vi "运维调试_五参数.vi"(11 "编号":string) -> ()   [LabVIEW 2016, in "斯坦道多参数.lvlib"]
uses:
  <vilib>/Utility/miscctls.llb/LVPointTypeDef.ctl
  <vilib>/Plasmionique/MB Master/MB_Master/MB_Master.lvclass
  <vilib>/Utility/config.llb/NI_LVConfig.lvlib
panel:
  in  "水样保存组数":dbl caption="水样保存组数:"
  in  "水样稳定时间":dbl caption="水样稳定时间:"
  in  "仪器参数":bool
  in  "参数设置选项卡":enum32{"选项卡 1", "选项卡 2"}(tab)
  in  "COD探头选择":u16(ring)=1 items=["YL型", "MQ型", "NAQ型"]
  in  "COD启用":bool
  in  "pH":bool
  in  "DO":bool
  in  "Turb":bool
  in  "Cond":bool
  in  "Temp":bool
  in  "叶绿素a启用":bool
  in  "藻密度":bool
  in  "pH探头选择":u16(ring) items=["YL型", "MQ型", "NAQ型"]
  in  "DO探头选择":u16(ring) items=["YL型", "MQ型", "NAQ型"]
  in  "电导率探头选择":u16(ring) items=["YL型", "MQ型", "NAQ型"]
  in  "浊度探头选择":u16(ring) items=["YL型", "MQ型", "NAQ型"]
  in  "叶绿素a探头选择":u16(ring) items=["YL型", "MQ型", "NAQ型"]
  in  "藻密度探头选择":u16(ring) items=["YL型", "MQ型", "NAQ型"]
  in  "ORP启用":bool
  in  "ORP探头选择":u16(ring) items=["YL型", "MQ型", "NAQ型"]
  in  "校准选择":T1
  out "模块版本号":string
  out "权限等级":string
  in  "打开modbus":bool
  out "选项卡控件":enum32{"选项卡 1", "选项卡 2"}(tab)
  in  "VISA资源名称":refnum<visa-resource-name> caption="串口"
  in  "IP":string="localhost" caption="IP:"
  in  "Port":u16=502 caption="Port:"
  in  "自动断线重连":bool=TRUE
  in  "连接方式":u16(ring) items=["Modbus RTU", "Modbus TCP"]
  in  "密码锁":bool
  in  "设置页返回":bool
  in  "周期设置":bool
  out "当前串口":string
  out "运行状态":enum16{"空闲", "水样测试", "标样核查"}(ring)
  in  "停止":bool
  in  "标样核查":bool
  in  "水样测试":bool
  in  "设置":bool
  in  "探头校正返回":bool
  in  "探头校正":bool
  out "检测值":T2
  # "请设置仪器连接方式"
  # "组"
  # "min"
  # "请选择要启用的参数"
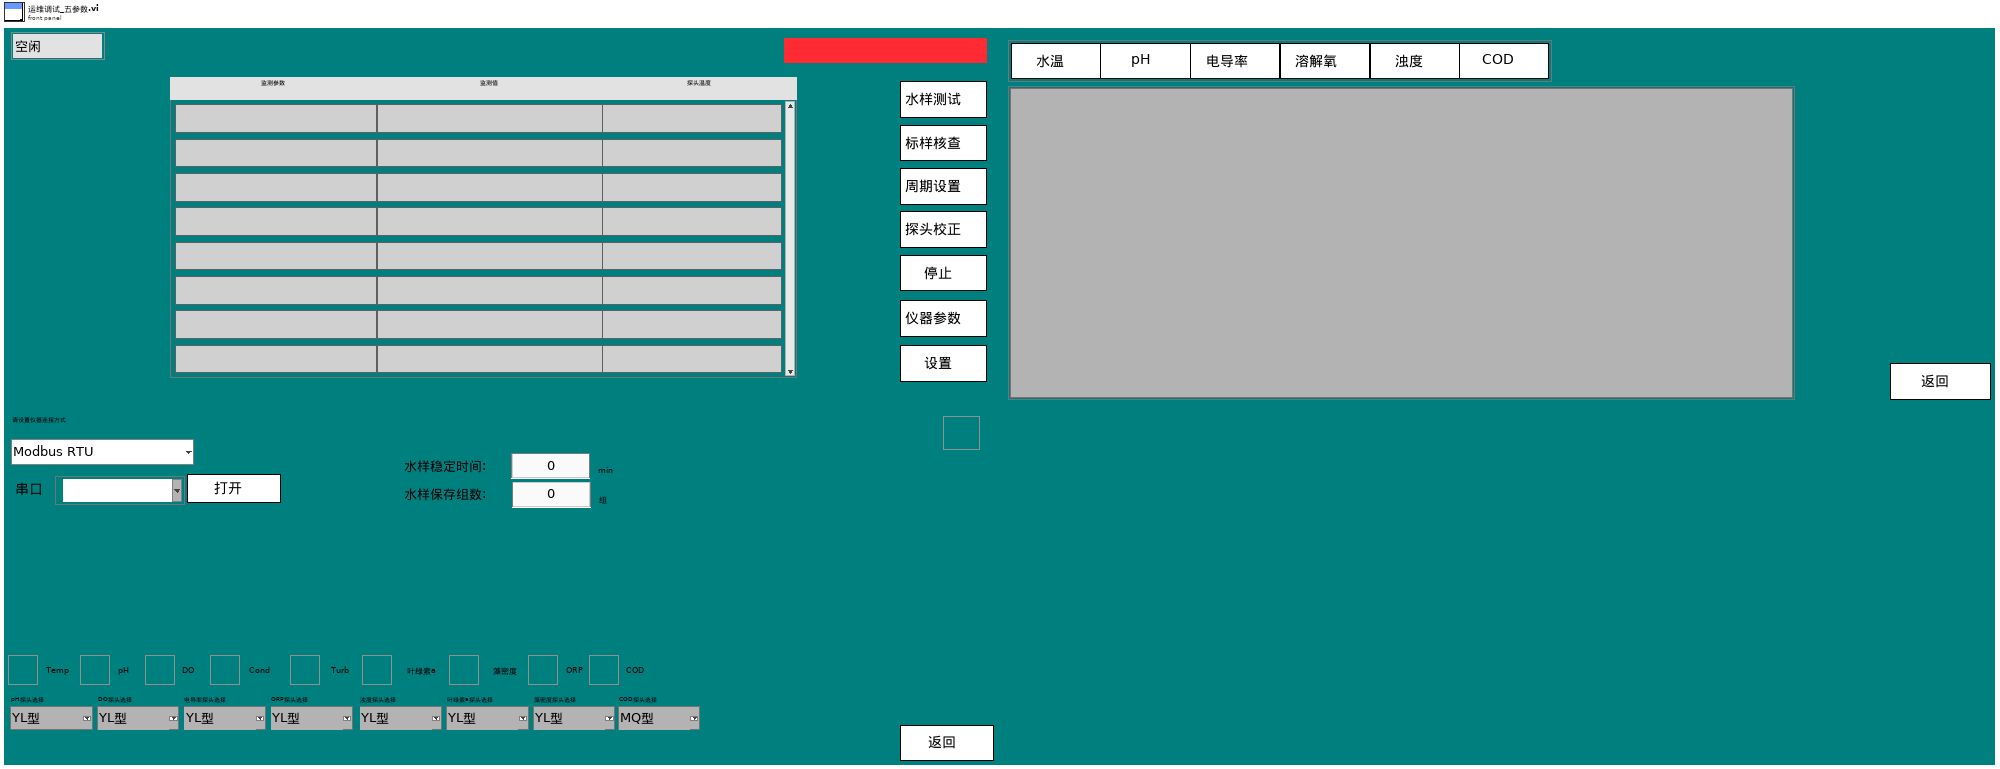
[diagram p1: front panel]
types:
  T1 = cluster{"水温校准":bool, "pH校准":bool, "电导率校准":bool, "溶解氧校准":bool, "浊度校准":bool, "叶绿素a校准":bool, "藻密度校准":bool, "ORP校准":bool, "COD校准":bool}
  T2 = typedef "斯坦道多参数.lvlib/检测值.ctl" = cluster{"监测参数1":string, "浓度1":string, "探头温度1":string}[]
  T3 = typedef "LVPointTypeDef.ctl" = cluster{"Horizontal":i16, "Vertical":i16}
  T4 = cluster{"CH":u16, "监测值":dbl, "温度偏移修正值":sgl, "信号值":sgl}
  T5 = cluster{"温度测量值":sgl, "测量值":sgl, "温度偏移修正值":sgl, "信号值":sgl}
  T6 = cluster{"温度测量值":sgl, "DO%":sgl, "DOmg/L":sgl, "温度偏移修正值":sgl}
  T7 = cluster{"电极状态标志":u16, "电极型号标志":u16, "浊度测量值":sgl, "温度测量值":sgl, "浊度信号值":sgl, "浊度偏移修正值":sgl, "温度偏移修正值":sgl, "手动温度补偿值":sgl, "浊度电极零点":sgl, "浊度电极斜率":sgl, "第1点标准值记录":sgl, "第1点信号值记录":sgl, "第1点温度值记录":sgl, "第2点标准值记录":sgl, "第2点信号值记录":sgl, "第2点温度值记录":sgl, "命令滤波设定":u16, "温度模式":enum16{"ATC", "MTC"}, "生产批次":u16, "电极序号":u16, "串口地址":u16, "串口波特率":enum16{"9600", "19200", "115200"}, "串口校验位":enum16{"NONE", "ODD", "EVEN"}, "串口停止位":enum16{"1bit", "2bit"}, "第一点标准值":sgl, "第二点标准值":sgl, "第三点标准值":sgl}
  T8 = cluster{"电极状态标志":u16, "电极型号标志":u16, "溶解氧测量值":sgl, "温度测量值":sgl, "溶解氧饱和度值":sgl, "盐度补偿值":sgl, "大气压补偿值":sgl, "溶解氧偏移修正值":sgl, "温度偏移修正值":sgl, "手动温度补偿值":sgl, "溶解氧电极零点":sgl, "溶解氧电极斜率":sgl, "第1点标准值记录":sgl, "第1点信号值记录":sgl, "第1点温度值记录":sgl, "第2点标准值记录":sgl, "第2点信号值记录":sgl, "第2点温度值记录":sgl, "命令滤波设定":u16, "温度模式":enum16{"ATC", "MTC"}, "生产批次":u16, "电极序号":u16, "串口地址":u16, "串口波特率":enum16{"9600", "19200", "115200"}, "串口校验位":enum16{"NONE", "ODD", "EVEN"}, "串口停止位":enum16{"1bit", "2bit"}, "第一点标准值":sgl, "第二点标准值":sgl}
  T9 = cluster{"电极状态标志":u16, "电极型号标志":u16, "酸碱度测量值":sgl, "温度测量值":sgl, "酸碱度信号值":sgl, "温度信号值":sgl, "酸碱度偏移修正值":sgl, "温度偏移修正值":sgl, "手动温度补偿值":sgl, "酸碱度电极零点":sgl, "酸碱度电极斜率":sgl, "第1点标准值记录":sgl, "第1点信号值记录":sgl, "第1点温度值记录":sgl, "第2点标准值记录":sgl, "第2点信号值记录":sgl, "第2点温度值记录":sgl, "命令滤波设定":u16, "温度模式":enum16{"ATC", "MTC"}, "生产批次":u16, "电极序号":u16, "串口地址":u16, "串口波特率":enum16{"9600", "19200", "115200"}, "串口校验位":enum16{"NONE", "ODD", "EVEN"}, "串口停止位":enum16{"1bit", "2bit"}, "第一点标准值":sgl, "第二点标准值":sgl}
  T10 = cluster{"测量量程":dbl, "测量精度":dbl, "测量间隔":dbl, "消解温度":dbl, "消解时长":dbl, "空白校准时间":timestamp, "曲线截距":dbl, "曲线斜率":dbl, "测量检出限":dbl, "测量信号值":dbl, "线性相关系数":dbl, "二次多项式系数":dbl, "标样校准时间":timestamp, "稀释倍数":dbl, "三项式系数":dbl, "空白标定系数":dbl, "量程系数":dbl, "F0/ORPA":dbl, "F1/ORPB":dbl, "F2/ORPK":dbl, "F3":dbl, "F4":dbl, "F5":dbl, "F6":dbl, "F7":dbl, "X0/滴定数":dbl, "量程":dbl}
  T11 = cluster{"电极状态标志":u16, "电极型号标志":u16, "电导率测量值":sgl, "温度测量值":sgl, "电导率信号值":sgl, "温度信号值":sgl, "温度补偿系数":sgl, "电导率偏移修正值":sgl, "温度偏移修正值":sgl, "手动温度补偿值":sgl, "电导率电极零点":sgl, "电导率电极斜率":sgl, "命令滤波设定":u16, "温度模式":enum16{"ATC", "MTC"}, "生产批次":u16, "电极序号":u16, "串口地址":u16, "串口波特率":enum16{"9600", "19200", "115200"}, "串口校验位":enum16{"NONE", "ODD", "EVEN"}, "串口停止位":enum16{"1bit", "2bit"}, "第一点标准值":sgl, "第二点标准值":sgl}
  T12 = enum8{"Enabled", "Disabled", "Disabled and Grayed Out"}
  T13 = cluster{"pH探头选择":u16, "DO探头选择":u16, "电导率探头选择":u16, "浊度探头选择":u16, "叶绿素a探头选择":u16, "蓝绿藻探头选择":u16, "orp探头选择":u16, "COD探头选择":u16}
  T14 = cluster{"监测参数1":string, "浓度1":string, "探头温度1":string}[]
  T15 = cluster{"周期设置类型":enum16{"定点启动", "间隔启动"}, "定时功能启用":bool, "定时间隔":u32, "24H周期设置":bool[]}
  T16 = enum32{"Bad", "Idle", "Run top level", "Running"}
  T17 = typedef "LVDateTimeRec.ctl" = cluster{"秒数的小数部分":dbl, "秒":i32, "分":i32, "时":i32, "日":i32, "月":i32, "年":i32, "天数（周）":i32, "天数（年）":i32, "DST":i32}
  T18 = cluster{"Major":u16, "Minor":u16, "Fix":u16, "Build":u16}
  T19 = typedef "NI_LVConfig.lvlib/Config Data RefNum.ctl" = refnum<k1>
  T20 = cluster{"baud rate (bps)":u32, "stop bits":u16, "parity":u16, "flow control":u16, "timeout":u32, "retries":i32}
  T21 = cluster{"pH校准VI引用句柄":refnum<vi>, "DO校准VI引用句柄":refnum<vi>, "COND校准VI引用句柄":refnum<vi>, "TURB校准VI引用句柄":refnum<vi>, "CHLA校准VI引用句柄":refnum<vi>, "BGA校准VI引用句柄":refnum<vi>, "ORP校准VI引用句柄":refnum<vi>, "COD校准VI引用句柄":refnum<vi>}
  T22 = cluster{"测量量程":dbl, "测量精度":dbl, "测量间隔":dbl, "消解温度":dbl, "消解时长":dbl, "空白校准时间":timestamp, "曲线截距":dbl, "曲线斜率":dbl, "测量检出限":dbl, "测量信号值":dbl, "线性相关系数":dbl, "二次多项式系数":dbl, "标样校准时间":timestamp, "稀释倍数":dbl, "三项式系数":dbl, "空白标定系数":dbl, "量程系数":dbl, "F0/ORPA":dbl, "F1/ORPB":dbl, "F2/ORPK":dbl, "F3":dbl, "F4":dbl, "F5":dbl, "F6":dbl, "F7":dbl, "X0/滴定数":dbl, "量程":dbl}[]
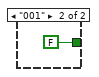
[diagram p3: hidden frame]
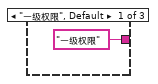
[diagram p12: hidden frame]
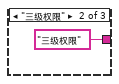
[diagram p13: hidden frame]
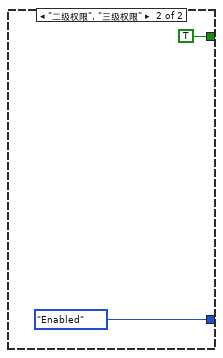
[diagram p14: hidden frame]
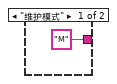
[diagram p19: hidden frame]
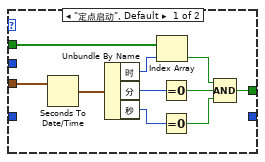
[diagram p20: hidden frame]
diagram:
  w34 = "data\\DCSset.ini" ("名称或相对路径")
  n1 = while {
    stop <- FALSE stop-if-true
    w64 = 0.0 ("二次多项式系数")
    n2 = global read "多参数全局变量.vi" "水温显示"() -> (w85:T4)
    n3 = global read "多参数全局变量.vi" "浊度显示"() -> (w67:T5)
    n4 = global read "多参数全局变量.vi" "DO显示"() -> (w99:T6)
    n5 = global read "多参数全局变量.vi" "ph显示"() -> (w94:T5)
    n6 = global read "国弘过程全局变量.vi" "Turb"() -> (w69:T7)
    n7 = Wait (ms)(milliseconds to wait=u32 1000 ("等待时间（毫秒）")) -> ()  [unwired: 1 out]
    n8 = global read "国弘过程全局变量.vi" "DO"() -> (w101:T8)
    n9 = global read "国弘过程全局变量.vi" "pH"() -> (w92:T9)
    n10 = Unbundle By Name(w101) -> ("溶解氧电极零点"=w102:sgl, "溶解氧电极斜率"=w103:sgl)
    n11 = Unbundle By Name(w92) -> ("酸碱度电极零点"=w91:sgl, "酸碱度电极斜率"=w90:sgl)
    n12 = Unbundle By Name(w69) -> ("浊度电极零点"=w70:sgl, "浊度电极斜率"=w71:sgl)
    n13 = Unbundle By Name(w85) -> ("信号值"=w86:sgl)
    n14 = Unbundle By Name(w67) -> ("信号值"=w68:sgl)
    n15 = Unbundle By Name(w94) -> ("信号值"=w93:sgl)
    n16 = Unbundle By Name(w99) -> ("DO%"=w100:sgl)
    n17 = global read "多参数全局变量.vi" "spcond显示"() -> (w80:T5)
    n18 = global read "断电保存变量.vi" "溶解氧参数"() -> (w97:T10)
    n19 = global read "断电保存变量.vi" "水温参数"() -> (w83:T10)
    n20 = global read "断电保存变量.vi" "浊度参数"() -> (w65:T10)
    n21 = global read "断电保存变量.vi" "PH参数"() -> (w96:T10)
    n22 = global read "国弘过程全局变量.vi" "Cond"() -> (w78:T11)
    n23 = Unbundle By Name(w78) -> ("电导率电极零点"=w77:sgl, "电导率电极斜率"=w76:sgl)
    n24 = Unbundle By Name(w80) -> ("信号值"=w79:sgl)
    n25 = global read "断电保存变量.vi" "电导率参数"() -> (w82:T10)
    n26 = Bundle By Name(cluster=w97, "测量信号值"=w100, "曲线截距"=w102, "曲线斜率"=w103, "线性相关系数"=1.0, "二次多项式系数"=0.0) -> (w98:T10)
    n27 = Bundle By Name(cluster=w65, "测量信号值"=w68, "曲线截距"=w70, "曲线斜率"=w71, "线性相关系数"=1.0, "二次多项式系数"=0.0) -> (w66:T10)
    n28 = Bundle By Name(cluster=w96, "测量信号值"=w93, "曲线截距"=w91, "曲线斜率"=w90, "线性相关系数"=1.0, "二次多项式系数"=0.0) -> (w95:T10)
    n29 = Bundle By Name(cluster=w83, "测量信号值"=w86, "曲线截距"=w64, "曲线斜率"=w64, "线性相关系数"=1.0, "二次多项式系数"=w64) -> (w84:T10)
    n30 = Bundle By Name(cluster=w82, "测量信号值"=w79, "曲线截距"=w77, "曲线斜率"=w76, "线性相关系数"=1.0, "二次多项式系数"=0.0) -> (w81:T10)
    n31 = global write "断电保存变量.vi" "溶解氧参数"(w98) -> ()
    n32 = global write "断电保存变量.vi" "水温参数"(w84) -> ()
    n33 = global write "断电保存变量.vi" "浊度参数"(w66) -> ()
    n34 = global write "断电保存变量.vi" "PH参数"(w95) -> ()
    n35 = global write "断电保存变量.vi" "电导率参数"(w81) -> ()
  }
  n36 = while {
    stop <- FALSE stop-if-true
    n37 = global read "多参数全局变量.vi" "多参数运行状态"() -> (→"运行状态":u16)
    n38 = Wait (ms)(milliseconds to wait=u32 1000 ("等待时间（毫秒）")) -> ()  [unwired: 1 out]
  }
  n39 = local read "编号"() -> (w10:string)
  n40 = call "程序默认配置.vi"() -> ()  [unwired: 11 in, 1 out]
  n41 = while {
    stop <- FALSE stop-if-true
    # "配置"
    n42 = global read "断电保存变量.vi" "Cond"() -> (w151:bool)
    n43 = global read "断电保存变量.vi" "Turb"() -> (w150:bool)
    n44 = global read "断电保存变量.vi" "Port"() -> (w129:u16)
    n45 = global read "断电保存变量.vi" "orp"() -> (w114:bool)
    n46 = global read "断电保存变量.vi" "DO"() -> (w152:bool)
    n47 = global read "断电保存变量.vi" "pH"() -> (w153:bool)
    n48 = global read "断电保存变量.vi" "IP"() -> (w130:string)
    n49 = global read "断电保存变量.vi" "水样测试组数"() -> (w112:dbl)
    n50 = global read "断电保存变量.vi" "连接方式"() -> (w122:u16)
    "选项卡控件" <- w122
    n51 = global read "断电保存变量.vi" "探头选择"() -> (w140:T13)
    n52 = Wait (ms)(milliseconds to wait=u32 500 ("等待时间（毫秒）")) -> ()  [unwired: 1 out]
    n53 = global read "断电保存变量.vi" "藻密度"() -> (w148:bool)
    n54 = global read "断电保存变量.vi" "Temp"() -> (w154:bool)
    n55 = local write "IP"(w130) -> ()
    n56 = local write "Turb"(w150) -> ()
    n57 = local write "Cond"(w151) -> ()
    n58 = local write "DO"(w152) -> ()
    n59 = local write "pH"(w153) -> ()
    n60 = local write "Port"(w129) -> ()
    n61 = local write "ORP启用"(w114) -> ()
    n62 = local write "连接方式"(w122) -> ()
    n63 = local write "Temp"(w154) -> ()
    n64 = Unbundle By Name(w140) -> ("orp探头选择"=w113:u16, "pH探头选择"=w123:u16, "DO探头选择"=w139:u16, "电导率探头选择"=w138:u16, "浊度探头选择"=w137:u16, "叶绿素a探头选择"=w136:u16, "蓝绿藻探头选择"=w135:u16)
    n65 = local write "藻密度"(w148) -> ()
    n66 = global read "多参数全局变量.vi" "MB session in"() -> (w144:refnum<class "MB_Master.lvclass">)
    n67 = local write "水样保存组数"(w112) -> ()
    n68 = global read "断电保存变量.vi" "VISA资源名称"() -> (w126:refnum<visa-resource-name>)
    n69 = global read "断电保存变量.vi" "自动断线重连"() -> (w117:bool)
    n70 = global read "断电保存变量.vi" "水样稳定时间"() -> (w116:dbl)
    n71 = global read "断电保存变量.vi" "叶绿素a启用"() -> (w149:bool)
    n72 = global read "断电保存变量.vi" "COD"() -> (w111:bool)
    n73 = global read "断电保存变量.vi" "连接方式"() -> (w127:u16)
    n74 = local write "COD启用"(w111) -> ()
    n75 = local write "自动断线重连"(w117) -> ()
    n76 = local write "ORP探头选择"(w113) -> ()
    n77 = local write "pH探头选择"(w123) -> ()
    n78 = local write "DO探头选择"(w139) -> ()
    n79 = local write "电导率探头选择"(w138) -> ()
    n80 = local write "浊度探头选择"(w137) -> ()
    n81 = local write "叶绿素a探头选择"(w136) -> ()
    n82 = local write "藻密度探头选择"(w135) -> ()
    n83 = local write "叶绿素a启用"(w149) -> ()
    n84 = global read "多参数全局变量.vi" "MB session in"() -> (w147:refnum<class "MB_Master.lvclass">)
    n85 = local write "水样稳定时间"(w116) -> ()
    n86 = local write "VISA资源名称"(w126) -> ()
    n87 = case shown="1" w127 {
      tunnel: w126 -> [w156 _]
      tunnel: [w156 w157] -> w125
      frame 0, Default {
      }
      frame 1 {
        n88 = global read "断电保存变量.vi" "Port"() -> (w158:u16)
        n89 = global read "断电保存变量.vi" "IP"() -> (w160:string)
        n90 = Format Into String(format string=":%d" ("格式字符串"), initial string=w160, w158) -> (resulting string=w157:string)  [unwired: 1 in, 1 out]
      }
    }
    "当前串口" <- w125
    n91 = property class="MB_Master"(reference=w144) -> ("Properties:Session Valid"=w121:bool)  [unwired: 1 in, 2 out]
    n92 = local read "密码锁"() -> (w134:bool)
    n93 = property class="MB_Master"(reference=w147) -> ("Properties:Session Valid"=w146:bool)  [unwired: 1 in, 2 out]
    n94 = Select(t=T12."Enabled" ("f"), s=w134, f=T12."Disabled") -> (s? t:f=w132:T12)
    n95 = Not(x=w121) -> (.not. x?=w124:bool)
    n96 = Select(t="关闭" ("布尔文本.文本"), s=w121, f="打开" ("布尔文本.文本")) -> (s? t:f=w141:string)
    n97 = Select(t=u32 16777216, s=w121, f=u32 16722483) -> (s? t:f=w118:u32)
    n98 = property on="当前串口" class="Str"("Blinking"=w124, "Text.BG Color"=w118) -> ()  [unwired: 2 in, 2 out]
    n99 = Select(t=T12."Disabled and Grayed Out" ("禁用"), s=w146, f=w132) -> (s? t:f=w128:T12)
    n100 = property on="IP" class="Str"("DisabledEnum"=w128) -> ()  [unwired: 2 in, 2 out]
    n101 = property on="Port" class="DigNum (严格)"("DisabledEnum"=w128) -> ()  [unwired: 2 in, 2 out]
    n102 = property on="VISA资源名称" class="VISAName"("DisabledEnum"=w128) -> ()  [unwired: 2 in, 2 out]
    n103 = property on="连接方式" class="Ring (严格)"("DisabledEnum"=w128) -> ()  [unwired: 2 in, 2 out]
    n104 = property on="打开modbus" class="Bool"("BoolText.Text"=w141) -> ()  [unwired: 2 in, 2 out]
  }
  n105 = vi-ref "水样测试.vi"() -> (w53:refnum<vi>)
  n106 = vi-ref "斯坦道多参数.lvlib:主副屏通信slave.vi"() -> (w35:refnum<vi>)
  n107 = control-ref of="本VI"() -> (w26:refnum<vi>)
  n108 = while {
    stop <- FALSE stop-if-true
    # "显示处理"
    n109 = global read "断电保存变量.vi" "Temp"() -> (w179:bool)
    n110 = Wait (ms)(milliseconds to wait=u32 1000 ("等待时间（毫秒）")) -> ()  [unwired: 1 out]
    n111 = case shown="真" w179 {
      tunnel: [w337 w342] -> w176
      tunnel: T14 [] ("数组") -> [w337 w343]
      tunnel: [T12."Disabled and Grayed Out" ("禁用") T12."Enabled" ("禁用")] -> _
      frame False {
      }
      frame True {
        n112 = global read "多参数全局变量.vi" "水温显示"() -> (w340:T4)
        n113 = Unbundle By Name(w340) -> ("CH"=w339:u16, "监测值"=w338:dbl)
        n114 = case shown="3" w339 {
          tunnel: ["水温 Temp (pH)" ("监测参数1") "水温 Temp (Cond)" ("监测参数1") "水温 Temp (DO)" ("监测参数1") "水温 Temp (Turb)" ("监测参数1")] -> w347
          frame 0, Default {
          }
          frame 1 {
          }
          frame 2 {
          }
          frame 3 {
          }
        }
        n115 = Format Into String(format string="%.2f ℃" ("格式字符串"), w338) -> (resulting string=w346:string)  [unwired: 2 in, 1 out]
        n116 = Bundle("监测参数1"=w347, w346, "探头温度1"="-") -> (w344:cluster{"监测参数1":string, string, "探头温度1":string})  [unwired: 1 in]
        n117 = Insert Into Array(array=w343, new element=w344) -> (w342:T14)  [unwired: 1 in]
      }
    }
    n118 = global read "断电保存变量.vi" "pH"() -> (w177:bool)
    n119 = case shown="真" w177 {
      tunnel: [w319 w327] -> w174
      tunnel: w176 -> [w319 w329]
      tunnel: [T12."Disabled and Grayed Out" ("禁用") T12."Enabled" ("禁用")] -> _
      frame False {
      }
      frame True {
        n120 = global read "多参数全局变量.vi" "ph显示"() -> (w325:T5)
        n121 = Unbundle By Name(w325) -> ("测量值"=w335:sgl, "信号值"=w320:sgl, "温度测量值"=w333:sgl)
        n122 = global read "多参数全局变量.vi" "ph通讯状态"() -> (w323:bool)
        n123 = Format Into String(format string="%.2f(%.2f mV)" ("格式字符串"), w335, w320) -> (resulting string=w322:string)  [unwired: 2 in, 1 out]
        n124 = Select(t="通讯异常" ("格式字符串"), s=w323, f=w322) -> (s? t:f=w321:string)
        n125 = Format Into String(format string="%.2f ℃" ("格式字符串"), w333) -> (resulting string=w331:string)  [unwired: 2 in, 1 out]
        n126 = Bundle("监测参数2"="酸碱度 pH", "格式字符串"=w321, w331) -> (w328:cluster{"监测参数2":string, "格式字符串":string, string})  [unwired: 1 in]
        n127 = Insert Into Array(array=w329, new element=w328) -> (w327:T14)  [unwired: 1 in]
      }
    }
    n128 = global read "断电保存变量.vi" "DO"() -> (w175:bool)
    n129 = case shown="真" w175 {
      tunnel: [w298 w305] -> w171
      tunnel: w174 -> [w298 w306]
      tunnel: [T12."Disabled and Grayed Out" ("禁用") T12."Enabled" ("禁用")] -> _
      frame False {
      }
      frame True {
        n130 = global read "多参数全局变量.vi" "DO显示"() -> (w303:T6)
        n131 = Unbundle By Name(w303) -> ("DOmg/L"=w314:sgl, "DO%"=w312:sgl, "温度测量值"=w316:sgl)
        n132 = global read "多参数全局变量.vi" "DO通讯状态"() -> (w301:bool)
        n133 = Format Into String(format string="%.2f mg/L" ("格式字符串"), w314) -> (resulting string=w311:string)  [unwired: 2 in, 1 out]
        n134 = Format Into String(format string="(%.2f %%)" ("格式字符串"), w312) -> (resulting string=w310:string)  [unwired: 2 in, 1 out]
        n135 = Concatenate Strings(w311, w310) -> (w300:string)
        n136 = Select(t="通讯异常" ("格式字符串"), s=w301, f=w300) -> (s? t:f=w299:string)
        n137 = Format Into String(format string="%.2f ℃" ("格式字符串"), w316) -> (resulting string=w308:string)  [unwired: 2 in, 1 out]
        n138 = Bundle("监测参数2"="溶解氧 DO", "格式字符串"=w299, w308) -> (w307:cluster{"监测参数2":string, "格式字符串":string, string})  [unwired: 1 in]
        n139 = Insert Into Array(array=w306, new element=w307) -> (w305:T14)  [unwired: 1 in]
      }
    }
    n140 = global read "断电保存变量.vi" "Cond"() -> (w173:bool)
    n141 = case shown="真" w173 {
      tunnel: w171 -> [w268 w292]
      tunnel: [w268 w281] -> w164
      tunnel: [T12."Disabled and Grayed Out" ("禁用") T12."Enabled" ("禁用")] -> _
      frame False {
      }
      frame True {
        n142 = global read "多参数全局变量.vi" "盐度显示"() -> (w274:T5)
        n143 = global read "多参数全局变量.vi" "spcond显示"() -> (w289:T5)
        n144 = Unbundle By Name(w274) -> ("测量值"=w275:sgl, "温度测量值"=w276:sgl)
        n145 = Unbundle By Name(w289) -> ("测量值"=w288:sgl, "温度测量值"=w287:sgl)
        n146 = global read "多参数全局变量.vi" "spcond通讯状态"() -> (w285:bool)
        n147 = global read "多参数全局变量.vi" "spcond通讯状态"() -> (w278:bool)
        n148 = Format Into String(format string="%.2f μS/cm" ("格式字符串"), w288) -> (resulting string=w284:string)  [unwired: 2 in, 1 out]
        n149 = Format Into String(format string="%.2f ppt" ("格式字符串"), w275) -> (resulting string=w279:string)  [unwired: 2 in, 1 out]
        n150 = Select(t="通讯异常" ("格式字符串"), s=w285, f=w284) -> (s? t:f=w283:string)
        n151 = Select(t="通讯异常" ("格式字符串"), s=w278, f=w279) -> (s? t:f=w280:string)
        n152 = Format Into String(format string="%.2f ℃" ("格式字符串"), w287) -> (resulting string=w293:string)  [unwired: 2 in, 1 out]
        n153 = Format Into String(format string="%.2f ℃" ("格式字符串"), w276) -> (resulting string=w273:string)  [unwired: 2 in, 1 out]
        n154 = Bundle("监测参数2"="电导率 Cond", "格式字符串"=w283, w293) -> (w291:cluster{"监测参数2":string, "格式字符串":string, string})  [unwired: 1 in]
        n155 = Insert Into Array(array=w292, new element=w291) -> (w282:T14)  [unwired: 1 in]
        n156 = Bundle("监测参数2"="盐度 Sal", "格式字符串"=w280, w273) -> (w269:cluster{"监测参数2":string, "格式字符串":string, string})  [unwired: 1 in]
        n157 = Insert Into Array(array=w282, new element=w269) -> (w281:T14)  [unwired: 1 in]
      }
    }
    n158 = global read "断电保存变量.vi" "orp"() -> (w166:bool)
    n159 = case shown="真" w166 {
      tunnel: w164 -> [w200 w211]
      tunnel: [w200 w209] -> w165
      tunnel: [T12."Disabled and Grayed Out" ("禁用") T12."Enabled" ("禁用")] -> _
      frame False {
      }
      frame True {
        n160 = global read "多参数全局变量.vi" "ORP显示"() -> (w207:T5)
        n161 = Unbundle By Name(w207) -> ("测量值"=w206:sgl, "温度测量值"=w205:sgl)
        n162 = global read "多参数全局变量.vi" "orp通讯状态"() -> (w203:bool)
        n163 = Format Into String(format string="%.2f mV" ("格式字符串"), w206) -> (resulting string=w202:string)  [unwired: 2 in, 1 out]
        n164 = Select(t="通讯异常" ("格式字符串"), s=w203, f=w202) -> (s? t:f=w201:string)
        n165 = Format Into String(format string="%.2f ℃" ("格式字符串"), w205) -> (resulting string=w212:string)  [unwired: 2 in, 1 out]
        n166 = Bundle("监测参数2"="ORP", "格式字符串"=w201, w212) -> (w210:cluster{"监测参数2":string, "格式字符串":string, string})  [unwired: 1 in]
        n167 = Insert Into Array(array=w211, new element=w210) -> (w209:T14)  [unwired: 1 in]
      }
    }
    n168 = global read "断电保存变量.vi" "Turb"() -> (w172:bool)
    n169 = case shown="真" w172 {
      tunnel: w165 -> [w251 w262]
      tunnel: [w251 w260] -> w170
      tunnel: [T12."Disabled and Grayed Out" ("禁用") T12."Enabled" ("禁用")] -> _
      frame False {
      }
      frame True {
        n170 = global read "多参数全局变量.vi" "浊度显示"() -> (w258:T5)
        n171 = Unbundle By Name(w258) -> ("测量值"=w257:sgl, "温度测量值"=w256:sgl)
        n172 = global read "多参数全局变量.vi" "浊度通讯状态"() -> (w254:bool)
        n173 = Format Into String(format string="%.2f NTU" ("格式字符串"), w257) -> (resulting string=w253:string)  [unwired: 2 in, 1 out]
        n174 = Select(t="通讯异常" ("格式字符串"), s=w254, f=w253) -> (s? t:f=w252:string)
        n175 = Format Into String(format string="%.2f ℃" ("格式字符串"), w256) -> (resulting string=w264:string)  [unwired: 2 in, 1 out]
        n176 = Bundle("监测参数2"="浊度 Turb", "格式字符串"=w252, w264) -> (w261:cluster{"监测参数2":string, "格式字符串":string, string})  [unwired: 1 in]
        n177 = Insert Into Array(array=w262, new element=w261) -> (w260:T14)  [unwired: 1 in]
      }
    }
    n178 = global read "断电保存变量.vi" "叶绿素a启用"() -> (w169:bool)
    n179 = case shown="真" w169 {
      tunnel: w170 -> [w234 w245]
      tunnel: [w234 w243] -> w167
      tunnel: [T12."Disabled and Grayed Out" ("禁用") T12."Enabled" ("禁用")] -> _
      frame False {
      }
      frame True {
        n180 = global read "多参数全局变量.vi" "叶绿素a显示"() -> (w239:T5)
        n181 = Unbundle By Name(w239) -> ("测量值"=w242:sgl, "温度测量值"=w241:sgl)
        n182 = global read "多参数全局变量.vi" "叶绿素a通讯状态"() -> (w237:bool)
        n183 = Format Into String(format string="%.2f μg/L" ("格式字符串"), w242) -> (resulting string=w236:string)  [unwired: 2 in, 1 out]
        n184 = Select(t="通讯异常" ("格式字符串"), s=w237, f=w236) -> (s? t:f=w235:string)
        n185 = Format Into String(format string="%.2f ℃" ("格式字符串"), w241) -> (resulting string=w247:string)  [unwired: 2 in, 1 out]
        n186 = Bundle("监测参数2"="叶绿素a Chla", "格式字符串"=w235, w247) -> (w244:cluster{"监测参数2":string, "格式字符串":string, string})  [unwired: 1 in]
        n187 = Insert Into Array(array=w245, new element=w244) -> (w243:T14)  [unwired: 1 in]
      }
    }
    n188 = global read "断电保存变量.vi" "藻密度"() -> (w168:bool)
    n189 = case shown="真" w168 {
      tunnel: w167 -> [w217 w228]
      tunnel: [w217 w226] -> w163
      tunnel: [T12."Disabled and Grayed Out" ("禁用") T12."Enabled" ("禁用")] -> _
      frame False {
      }
      frame True {
        n190 = global read "多参数全局变量.vi" "藻密度显示"() -> (w222:T5)
        n191 = Unbundle By Name(w222) -> ("测量值"=w225:sgl, "温度测量值"=w224:sgl)
        n192 = global read "多参数全局变量.vi" "藻密度通讯状态"() -> (w220:bool)
        n193 = Format Into String(format string="%.2f cells/mL" ("格式字符串"), w225) -> (resulting string=w219:string)  [unwired: 2 in, 1 out]
        n194 = Select(t="通讯异常" ("格式字符串"), s=w220, f=w219) -> (s? t:f=w218:string)
        n195 = Format Into String(format string="%.2f ℃" ("格式字符串"), w224) -> (resulting string=w230:string)  [unwired: 2 in, 1 out]
        n196 = Bundle("监测参数2"="藻密度 Algal", "格式字符串"=w218, w230) -> (w227:cluster{"监测参数2":string, "格式字符串":string, string})  [unwired: 1 in]
        n197 = Insert Into Array(array=w228, new element=w227) -> (w226:T14)  [unwired: 1 in]
      }
    }
    n198 = global read "断电保存变量.vi" "COD"() -> (w161:bool)
    n199 = case shown="真" w161 {
      tunnel: w163 -> [w183 w194]
      tunnel: [w183 w192] -> w162
      tunnel: [T12."Disabled and Grayed Out" ("禁用") T12."Enabled" ("禁用")] -> _
      frame False {
      }
      frame True {
        n200 = global read "多参数全局变量.vi" "COD显示"() -> (w188:T5)
        n201 = Unbundle By Name(w188) -> ("测量值"=w191:sgl, "温度测量值"=w190:sgl)
        n202 = global read "多参数全局变量.vi" "cod通讯状态"() -> (w186:bool)
        n203 = Format Into String(format string="%.2f mg/L" ("格式字符串"), w191) -> (resulting string=w185:string)  [unwired: 2 in, 1 out]
        n204 = Select(t="通讯异常" ("格式字符串"), s=w186, f=w185) -> (s? t:f=w184:string)
        n205 = Format Into String(format string="%.2f ℃" ("格式字符串"), w190) -> (resulting string=w196:string)  [unwired: 2 in, 1 out]
        n206 = Bundle("监测参数2"="COD", "格式字符串"=w184, w196) -> (w193:cluster{"监测参数2":string, "格式字符串":string, string})  [unwired: 1 in]
        n207 = Insert Into Array(array=w194, new element=w193) -> (w192:T14)  [unwired: 1 in]
      }
    }
    "检测值" <- w162
  }
  n208 = while {
    shift-right: [w376] -> _
    shift-left: u32 0 ("等待时间（毫秒）") -> [w377]
    stop <- FALSE stop-if-true
    # "密码权限"
    n209 = global read "多参数全局变量.vi" "权限"() -> (w367:enum16{"一级权限", "二级权限", "三级权限"})
    n210 = global read "多参数全局变量.vi" "权限"() -> (w368:enum16{"一级权限", "二级权限", "三级权限"})
    n211 = global read "多参数全局变量.vi" "权限"() -> (w369:enum16{"一级权限", "二级权限", "三级权限"})
    n212 = local read "连接方式"() -> (w373:u16)
    n213 = local read "密码锁"() -> (w378:bool)
    n214 = Wait (ms)(milliseconds to wait=u32 1000 ("等待时间（毫秒）")) -> ()  [unwired: 1 out]
    n215 = case shown="\"一级权限\", 默认" w367 {
      tunnel: [T12."Disabled" ("禁用") T12."Enabled" ("禁用")] -> w371
      tunnel: [_ TRUE ("可见")] -> w366
      frame "一级权限", Default {
      }
      frame "二级权限", "三级权限" {
      }
    }
    n216 = case shown="\"三级权限\"" w368 {
      tunnel: [_ TRUE ("可见")] -> w354
      frame "一级权限", Default {
      }
      frame "三级权限" {
      }
    }
    n217 = case shown="\"二级权限\"" w369 {
      tunnel: ["一级权限" ("权限等级") "三级权限" ("权限等级") "二级权限" ("权限等级")] -> w370
      frame "一级权限", Default {
      }
      frame "三级权限" {
      }
      frame "二级权限" {
      }
    }
    "权限等级" <- w370
    n218 = global read "断电保存变量.vi" "叶绿素a启用"() -> (w358:bool)
    n219 = global read "断电保存变量.vi" "藻密度"() -> (w357:bool)
    n220 = global read "断电保存变量.vi" "Temp"() -> (w364:bool)
    n221 = case shown="真" w378 {
      tunnel: w377 -> [_ w386]
      tunnel: [_ w385] -> w376
      frame False {
      }
      frame True {
        n222 = Increment(x=w386) -> (x+1=w385:u32)
      }
    }
    n223 = case shown="1" w373 {
      tunnel: [_ TRUE ("可见")] -> w372
      frame 0, Default {
      }
      frame 1 {
      }
    }
    n224 = global read "断电保存变量.vi" "Cond"() -> (w361:bool)
    n225 = global read "断电保存变量.vi" "COD"() -> (w353:bool)
    n226 = global read "断电保存变量.vi" "Turb"() -> (w359:bool)
    n227 = global read "断电保存变量.vi" "orp"() -> (w356:bool)
    n228 = global read "断电保存变量.vi" "DO"() -> (w360:bool)
    n229 = global read "断电保存变量.vi" "pH"() -> (w362:bool)
    n230 = property on="校准选择" class="Clust"() -> ("Controls[]"=w365:refnum<vi>[])  [unwired: 2 in, 2 out]
    n231 = Insert Into Array(array=bool[] [] ("数组"), new element #1=w364, new element #2=w362, new element #3=w361, new element #4=w360, new element #5=w359, new element #6=w358, new element #7=w357, new element #8=w356, new element #9=w353) -> (w355:bool[])  [unwired: 1 in]
    n232 = for {
      tunnel: w365 -> [w382] mode=indexing
      tunnel: w355 -> [w381] mode=indexing
      n233 = property class="Ctl"(reference=w382, "Visible"=w381) -> ()  [unwired: 1 in, 2 out]
    }
    n234 = property on="参数设置选项卡" class="TabCtl (严格)"("Visible"=w354) -> ()  [unwired: 2 in, 2 out]
    n235 = property on="自动断线重连" class="Bool (严格)"("Visible"=w372) -> ()  [unwired: 2 in, 2 out]
    n236 = Greater Or Equal?(x=w376, y=u32 1800) -> (x >= y?=w374:bool)
    n237 = local write "密码锁"(w366) -> ()
    n238 = property on="自动断线重连" class="Bool (严格)"("DisabledEnum"=w371) -> ()  [unwired: 2 in, 2 out]
    n239 = property on="打开modbus" class="Bool"("DisabledEnum"=w371) -> ()  [unwired: 2 in, 2 out]
    n240 = case shown="真" w374 {
      frame False {
      }
      frame True {
        n241 = global write "多参数全局变量.vi" "权限"(enum16{"一级权限", "二级权限", "三级权限"}."一级权限" ("权限")) -> ()
      }
    }
  }
  n242 = while {
    tunnel: w53 -> [w396]
    shift-right: [w395] -> _
    shift-left: u32 0 ("等待时间（毫秒）") -> [w397]
    stop <- FALSE stop-if-true
    # "周期控制"
    n243 = global read "断电保存变量.vi" "定时控制输入"() -> (w399:T15)
    n244 = Wait (ms)(milliseconds to wait=u32 500 ("等待时间（毫秒）")) -> ()  [unwired: 1 out]
    n245 = Unbundle By Name(w399) -> ("周期设置类型"=w401:enum16{"定点启动", "间隔启动"}, "24H周期设置"=w400:bool[], "定时间隔"=w398:u32, "定时功能启用"=w394:bool)
    n246 = case shown="真" w394 {
      tunnel: w401 -> [_ w412]
      tunnel: w400 -> [_ w411]
      tunnel: w398 -> [_ w409]
      tunnel: w397 -> [_ w405]
      tunnel: w396 -> [_ w408]
      tunnel: [_ w404] -> w395
      frame False {
      }
      frame True {
        n247 = property class="VI"(reference=w408) -> ("Exec.State"=w406:T16, "Name"=w407:string)  [unwired: 1 in, 2 out]
        n248 = Get Date/Time In Seconds() -> (seconds since 1Jan1904=w413:timestamp)
        n249 = case shown="\"间隔启动\"" w412 {
          tunnel: w413 -> [w435 _]
          tunnel: w411 -> [w432 _]
          tunnel: [w426 w443] -> w410
          tunnel: w409 -> [_ w442]
          tunnel: w405 -> [_ w444]
          tunnel: [_ w438] -> w404
          frame "定点启动", Default {
            n250 = Seconds To Date/Time(time stamp (now)=w435) -> (date time rec=w434:T17)  [unwired: 1 in]
            n251 = Unbundle By Name(w434) -> ("时"=w433:i32, "分"=w431:i32, "秒"=w430:i32)
            n252 = Index Array(array=w432, index=w433) -> (element=w429:bool)
            n253 = Equal To 0?(x=w431) -> (x = 0?=w428:bool)
            n254 = Equal To 0?(x=w430) -> (x = 0?=w427:bool)
            n255 = Compound Arithmetic op=AND ("复合运算")(w429, w428, w427) -> (w426:bool)
          }
          frame "间隔启动" {
            n256 = Increment(x=w444) -> (x+1=w437:u32)
            n257 = Multiply(x=w442, y=u32 120) -> (x*y=w436:u32)
            n258 = Less?(x=w436, y=w437) -> (x < y?=w440:bool)
            n259 = Select(t=u32 0 ("y"), s=w440, f=w437) -> (s? t:f=w438:u32)
            n260 = Equal To 0?(x=w444) -> (x = 0?=w443:bool)
          }
        }
        n261 = case shown="真" w410 {
          tunnel: w406 -> [_ w415]
          tunnel: w407 -> [_ w414]
          frame False {
          }
          frame True {
            n262 = case shown="\"Idle\"" w415 {
              tunnel: w414 -> [_ w420]
              frame "Bad", Default {
              }
              frame "Idle" {
                n263 = global read "多参数全局变量.vi" "运行模式"() -> (w418:enum16{"维护模式", "常规模式", "应急模式", "质控模式"})
                n264 = case shown="\"常规模式\", 默认" w418 {
                  tunnel: ["M" ("数据标记表") "N" ("数据标记表")] -> w417
                  frame "维护模式" {
                  }
                  frame "常规模式", Default {
                  }
                }
                n265 = Open VI Reference(type specifier VI Refnum (for type only)=refnum<vi> refnum, vi path=w420, options=128 ("选项")) -> (vi reference=w421:refnum<vi>)  [unwired: 3 in, 1 out]
                n266 = call-by-ref "开始异步调用"(reference=w421, "数据标记表"=w417) -> (reference out=w422:refnum<vi>, error out=w423:errorcluster)  [unwired: 12 in]
                n267 = Close Reference(reference=w422, error in (no error)=w423) -> ()  [unwired: 1 out]
              }
            }
          }
        }
      }
    }
    n268 = local write "周期设置"(w394) -> ()
  }
  n269 = property class="VI"(reference=w26) -> ("Library.Version"=w25:T18)  [unwired: 1 in, 2 out]
  n270 = Equal?(x=w10, y="") -> (x = y?=w12:bool)
  n271 = String To IP(1:"192.168.1.100" ("名称")) -> (0:w33:u32)
  n272 = IP To String(1:TRUE ("句点符号？(F)"), 2:w33) -> (0:w30:string)
  n273 = Select(t="1", s=w12, f=w10) -> (s? t:f=w9:string)
  n274 = Unbundle By Name(w25) -> ("Major"=w23:u16, "Minor"=w22:u16, "Fix"=w21:u16, "Build"=w20:u16)
  n275 = call "探头数据读取.vi"("编号"=w9) -> ()  [unwired: 11 in]
  n276 = Concatenate Strings("\\\\" ("字符串"), w30) -> (w31:string)
  n277 = Format Into String(format string="模块版本号：%d.%d.%d.%d" ("格式字符串"), w23, w22, w21, w20) -> (resulting string=→"模块版本号":string)  [unwired: 2 in, 1 out]
  n278 = property class="VI"(reference=w35, error in=errorcluster {"status"=FALSE, "code"=0, "source"=""} ("错误输出")) -> ("Name"=w36:string)  [unwired: 2 out]
  n279 = String To Path(string=w31) -> (path=w28:path)
  n280 = Open VI Reference(type specifier VI Refnum (for type only)=refnum<vi> refnum, vi path=w36, options=128 ("选项")) -> (vi reference=w38:refnum<vi>, error out=w40:errorcluster)  [unwired: 3 in]
  n281 = Build Path(base path=w28, name or relative path=w34) -> (appended path=w4:path)
  n282 = call-by-ref "?"(reference=w38, error in=w40) -> (reference out=w42:refnum<vi>, error out=w41:errorcluster)  [unwired: 12 in]
  n283 = global read "多参数全局变量.vi" "TCP Connection Count"() -> (w5:u32)
  n284 = Close Reference(reference=w42, error in (no error)=w41) -> ()  [unwired: 1 out]
  n285 = case shown="1, 默认" w5 {
    tunnel: w4 -> [w445 w448]
    tunnel: [w445 w447] -> w2
    tunnel: [_ w446] -> w3
    frame 0 {
    }
    frame 1, Default {
      n286 = call <vilib>:"Check if File or Folder Exists.vi"("path"=w448) -> ("file or folder exists?"=w446:bool, "dup path"=w447:path)  [unwired: 8 in, 1 out]
    }
  }
  n287 = case shown="假" w3 {
    tunnel: w2 -> [_ w452]
    tunnel: [w450 w452] -> w7
    tunnel: w34 -> [w449 _]
    frame False {
      # "本地文件地址"
      n288 = call <vilib>:"Application Directory.vi"() -> ("Application Directory"=w451:path)
      n289 = Build Path(base path=w451, name or relative path=w449) -> (appended path=w450:path)
    }
    frame True {
      # "网络共享地址"
    }
  }
  n290 = global write "多参数全局变量.vi" "配置文件 path"(w7) -> ()
  n291 = Equal?(x="编号", y="") -> (x = y?=w17:bool)
  n292 = call <vilib>:"Open Config Data.vi"("configuration file path"=w7) -> ("error out"=w47:errorcluster, "refnum"=w48:T19)  [unwired: 8 in, 1 out]
  n293 = Select(t="1", s=w17, f="编号") -> (s? t:f=w15:string)
  n294 = global write "多参数全局变量.vi" "多参数编号"(w15) -> ()
  n295 = vi-ref "断电保存变量.vi"() -> (w44:refnum<vi>)
  n296 = case shown="\"假\", 默认" w15 {
    tunnel: [TRUE ("可见") FALSE ("可见")] -> w27
    frame "假", Default {
    }
    frame "001" {
    }
  }
  n297 = Concatenate Strings("MPresource" ("名称（未命名）"), w15) -> (w55:string)
  n298 = call <userlib>:"Read Panel from INI__ogtk.vi"("error in (no error)"=w47, "VI ref"=w44, "refnum"=w48) -> ("error out"=w45:errorcluster, "refnum out"=w46:T19)  [unwired: 7 in]
  n299 = Concatenate Strings("MPP" ("名称（未命名）"), w15) -> (w56:string)
  n300 = call <vilib>:"Close Config Data.vi"("error in (no error)"=w45, "refnum"=w46) -> ("error out"=w8:errorcluster)  [unwired: 8 in, 1 out]
  n301 = Obtain Queue(name (unnamed)=w55, element data type="" ("名称（未命名）")) -> (queue out=w51:refnum<queue>)  [unwired: 3 in, 2 out]
  n302 = property on="窗格" class="Pane"("Origin"=T3 {"Horizontal"=0, "Vertical"=0} ("原点")) -> (error out=w63:errorcluster)  [unwired: 2 in, 1 out]
  n303 = Read from Text File(file (use dialog)=w7, error in=w8) -> (error out=w6:errorcluster)  [unwired: 2 in, 3 out]
  n304 = Obtain Notifier(name (unnamed)=w56, notification data type=FALSE) -> (notifier out=w59:refnum<notifier>)  [unwired: 2 in, 2 out]
  n305 = Enqueue Element(queue=w51, element="open" ("元素")) -> (queue out=w50:refnum<queue>)  [unwired: 2 in, 2 out]
  n306 = while {
    tunnel: [w462] -> _
    shift-right: [w455] -> _
    shift-left: _ -> [w460]
    tunnel: w6 -> [w457]
    stop <- FALSE stop-if-true
    n307 = Wait (ms)(milliseconds to wait=u32 1000 ("等待时间（毫秒）")) -> ()  [unwired: 1 out]
    n308 = global read "多参数全局变量.vi" "配置文件 path"() -> (w456:path)
    n309 = File/Directory Info(path=w456, error in=w457) -> (last mod=w455:timestamp, error out=w458:errorcluster)  [unwired: 5 out]
    n310 = Not Equal?(x=w455, y=w460) -> (x != y?=w459:bool)
    n311 = case shown="真" w459 {
      tunnel: [w464 w472] -> w462
      tunnel: w458 -> [w464 w471]
      tunnel: w456 -> [_ w465]
      frame False {
      }
      frame True {
        # "文件发生改变进行更新"
        n312 = call <vilib>:"Open Config Data.vi"("error in (no error)"=w471, "configuration file path"=w465) -> ("error out"=w470:errorcluster, "refnum"=w469:T19)  [unwired: 7 in, 1 out]
        n313 = vi-ref "断电保存变量.vi"() -> (w466:refnum<vi>)
        n314 = call <userlib>:"Read Panel from INI__ogtk.vi"("error in (no error)"=w470, "VI ref"=w466, "refnum"=w469) -> ("error out"=w468:errorcluster, "refnum out"=w467:T19)  [unwired: 7 in]
        n315 = call <vilib>:"Close Config Data.vi"("error in (no error)"=w468, "refnum"=w467) -> ("error out"=w472:errorcluster)  [unwired: 8 in, 1 out]
      }
    }
  }
  n316 = while {
    tunnel: w50 -> [w474]
    tunnel: w6 -> [_]
    stop <- FALSE stop-if-true
    n317 = Dequeue Element(queue=w474) -> (element=w473:string)  [unwired: 2 in, 3 out]
    n318 = case shown="\"open\"" w473 {
      tunnel: [_ w476 w486] -> _
      frame "假", Default {
      }
      frame "open" {
        n319 = global read "多参数全局变量.vi" "MB session in"() -> (w481:refnum<class "MB_Master.lvclass">)
        n320 = global read "断电保存变量.vi" "VISA资源名称"() -> (w483:refnum<visa-resource-name>)
        n321 = global read "断电保存变量.vi" "连接方式"() -> (w479:u16)
        n322 = call "close MB.vi"("MB session in"=w481) -> ("error out"=w484:errorcluster)  [unwired: 10 in]
        n323 = global read "断电保存变量.vi" "Port"() -> (w477:u16)
        n324 = global read "断电保存变量.vi" "IP"() -> (w478:string)
        n325 = call "open MB.vi"("Port (502)"=w477, "IP Address"=w478, "MODE"=w479, "error in (no error)"=w484, "Serial Config"=T20 {"baud rate (bps)"=9600, "stop bits"=10, "parity"=0, "flow control"=0, "timeout"=1000, "retries"=1}, "VISA资源名称"=w483) -> ("error out"=w476:errorcluster, "MB session out"=w480:refnum<class "MB_Master.lvclass">)  [unwired: 4 in]
        n326 = global write "多参数全局变量.vi" "MB session in"(w480) -> ()
      }
      frame "close" {
        n327 = global read "多参数全局变量.vi" "MB session in"() -> (w485:refnum<class "MB_Master.lvclass">)
        n328 = call "close MB.vi"("MB session in"=w485) -> ("error out"=w486:errorcluster)  [unwired: 10 in]
      }
    }
  }
  n329 = while {
    tunnel: w50 -> [w488]
    stop <- FALSE stop-if-true
    # "断线重连"
    n330 = global read "断电保存变量.vi" "连接方式"() -> (w489:u16)
    n331 = Wait (ms)(milliseconds to wait=u32 10000 ("等待时间（毫秒）")) -> ()  [unwired: 1 out]
    n332 = case shown="1" w489 {
      tunnel: w488 -> [_ w492]
      frame 0, Default {
      }
      frame 1 {
        n333 = case shown="真" "自动断线重连" {
          tunnel: w492 -> [_ w495]
          frame False {
          }
          frame True {
            n334 = global read "多参数全局变量.vi" "MB session in"() -> (w494:refnum<class "MB_Master.lvclass">)
            n335 = property class="MB_Master"(reference=w494) -> ("Properties:Session Valid"=w493:bool)  [unwired: 1 in, 2 out]
            n336 = case shown="假" w493 {
              tunnel: w495 -> [w496 _]
              frame False {
                n337 = Flush Queue(queue=w496) -> (queue out=w498:refnum<queue>)  [unwired: 1 in, 2 out]
                n338 = Enqueue Element(queue=w498, element="open" ("元素")) -> ()  [unwired: 2 in, 3 out]
              }
              frame True {
              }
            }
          }
        }
      }
    }
  }
  n339 = while {
    tunnel: w63 -> [_]
    tunnel: w59 -> [w500]
    tunnel: w50 -> [w499]
    stop <- FALSE stop-if-true
    n340 = event shown="[9] \"标样核查\": 值改变" {
      selector: _ -> [_ _ _ _ _ _ _ _ _ _ _ _ _ _ _ _ _ _ _ _ _ _ _ _ _]
      dyn-events: _ -> [_ _ _ _ _ _ _ _ _ _ _ _ _ _ _ _ _ _ _ _ _ _ _ _ _]
      timeout: _ -> [_ _ _ _ _ _ _ _ _ _ _ _ _ _ _ _ _ _ _ _ _ _ _ _ _]
      tunnel: w500 -> [_ _ _ _ _ _ _ _ _ _ w608 _ _ _ _ _ _ _ _ _ _ _ _ _ _]
      tunnel: w499 -> [_ _ _ _ _ _ _ _ _ _ _ _ _ _ w648 _ _ _ _ _ _ _ _ _ _]
      event Timeout {
        n341 = event-data() -> ()  [unwired: 1 in, 3 out]
      }
      event "水样稳定时间", "水样保存组数": Mouse Down {
        n342 = event-data() -> ("CtlRef"=w502:refnum<vi>)  [unwired: 1 in, 7 out]
        n343 = property class="DigNum (严格)"(reference=w502) -> (reference out=w505:refnum<vi>, "Value"=w504:dbl)  [unwired: 1 in, 1 out]
        n344 = call "数字键盘.vi"("OldNumber"=w504) -> ("NewNumber"=w503:dbl)  [unwired: 1 in]
        n345 = property class="DigNum (严格)"(reference=w505, "Val(Sgnl)"=w503) -> ()  [unwired: 1 in, 2 out]
      }
      event "pH探头选择", "DO探头选择", "电导率探头选择", "浊度探头选择", "叶绿素a探头选择", "藻密度探头选择", "ORP探头选择", "COD探头选择": Value Change {
        n346 = event-data() -> ("CtlRef"=w506:refnum<vi>, "NewVal"=w507:u16)  [unwired: 1 in, 4 out]
        n347 = Two Button Dialog(message="请再次确认修改的型号是否与实际匹配，否则将导致通讯异常，并且此操作将终止所有正在校准的参数！" ("消息")) -> (T button?=w508:bool)  [unwired: 2 in]
        n348 = case shown="真" w508 {
          tunnel: w507 -> [_ w511]
          tunnel: w506 -> [_ w510]
          frame False {
          }
          frame True {
            n349 = flat-sequence {
              tunnel: w511 -> [w512]
              tunnel: w510 -> [w516]
              frame #0 {
                n350 = property class="Ring (严格)"(reference=w516) -> ("Label.Text"=w515:string)  [unwired: 1 in, 2 out]
                n351 = global read "断电保存变量.vi" "探头选择"() -> (w514:T13)
                n352 = global read "多参数全局变量.vi" "校准VI引用句柄"() -> (w517:T21)
                n353 = case shown="\"COD探头选择\"" w515 {
                  tunnel: w514 -> [w519 w522 w525 w528 w531 w534 w537 w540 w543]
                  tunnel: [w519 w521 w524 w527 w530 w533 w536 w539 w542] -> w513
                  tunnel: w512 -> [_ w520 w523 w526 w529 w532 w535 w538 w541]
                  frame Default {
                  }
                  frame "pH探头选择" {
                    n354 = Bundle By Name(cluster=w522, "pH探头选择"=w520) -> (w521:T13)
                  }
                  frame "电导率探头选择" {
                    n355 = Bundle By Name(cluster=w525, "电导率探头选择"=w523) -> (w524:T13)
                  }
                  frame "DO探头选择" {
                    n356 = Bundle By Name(cluster=w528, "DO探头选择"=w526) -> (w527:T13)
                  }
                  frame "浊度探头选择" {
                    n357 = Bundle By Name(cluster=w531, "浊度探头选择"=w529) -> (w530:T13)
                  }
                  frame "叶绿素a探头选择" {
                    n358 = Bundle By Name(cluster=w534, "叶绿素a探头选择"=w532) -> (w533:T13)
                  }
                  frame "蓝绿藻探头选择" {
                    n359 = Bundle By Name(cluster=w537, "蓝绿藻探头选择"=w535) -> (w536:T13)
                  }
                  frame "ORP探头选择" {
                    n360 = Bundle By Name(cluster=w540, "orp探头选择"=w538) -> (w539:T13)
                  }
                  frame "COD探头选择" {
                    n361 = Bundle By Name(cluster=w543, "COD探头选择"=w541) -> (w542:T13)
                  }
                }
                n362 = Cluster To Array(cluster=w517) -> (array=w518:refnum<vi>[])
                n363 = for {
                  tunnel: w518 -> [w545] mode=indexing
                  tunnel: [w544] -> _ mode=indexing
                  n364 = invoke class="VI" method="Abort VI"(reference=w545) -> (error out=w544:errorcluster)  [unwired: 2 in, 2 out]
                }
                n365 = global write "断电保存变量.vi" "探头选择"(w513) -> ()
              }
              frame #1 {
                n366 = call "配置文件保存.vi"() -> ()  [unwired: 12 in]
              }
            }
          }
        }
      }
      event "VISA资源名称", "pH", "DO", "Turb", "Cond", "Temp", "叶绿素a启用", "打开modbus", "藻密度", "连接方式", "自动断线重连", "ORP启用": Mouse Down {
        n367 = event-data() -> ()  [unwired: 1 in, 6 out]
        n368 = local read "密码锁"() -> (w546:bool)
        n369 = case shown="假" w546 {
          frame False {
            n370 = One Button Dialog(message="当前操作权限不足,请提升权限!!!" ("消息")) -> ()  [unwired: 1 in, 1 out]
          }
          frame True {
          }
        }
      }
      event "IP": Mouse Down {
        n371 = event-data() -> ("CtlRef"=w549:refnum<vi>)  [unwired: 1 in, 7 out]
        n372 = property on="IP" class="Str"() -> ("DisabledEnum"=w548:T12)  [unwired: 2 in, 2 out]
        n373 = case shown="\"Disabled and Grayed Out\"" w548 {
          tunnel: w549 -> [w553 _ _]
          frame "Enabled" {
            n374 = property class="Str"(reference=w553) -> (reference out=w552:refnum<vi>, "Value"=w551:string)  [unwired: 1 in, 1 out]
            n375 = call "字符键盘.vi"("Old String"=w551) -> ("String"=w550:string)  [unwired: 10 in]
            n376 = property class="Str"(reference=w552, "Val(Sgnl)"=w550) -> ()  [unwired: 1 in, 2 out]
          }
          frame "Disabled and Grayed Out" {
            n377 = One Button Dialog(message="关闭连接后才可设置!" ("消息")) -> ()  [unwired: 1 in, 1 out]
          }
          frame "Disabled", Default {
            n378 = One Button Dialog(message="当前操作权限不足,请提升权限!!!" ("消息")) -> ()  [unwired: 1 in, 1 out]
          }
        }
      }
      event "Port": Mouse Down {
        n379 = event-data() -> ("CtlRef"=w557:refnum<vi>)  [unwired: 1 in, 7 out]
        n380 = property on="Port" class="DigNum (严格)"() -> ("DisabledEnum"=w556:T12)  [unwired: 2 in, 2 out]
        n381 = case shown="\"Enabled\"" w556 {
          tunnel: w557 -> [w561 _ _]
          frame "Enabled" {
            n382 = property class="DigNum (严格)"(reference=w561) -> (reference out=w560:refnum<vi>, "Value"=w559:u16)  [unwired: 1 in, 1 out]
            n383 = call "数字键盘.vi"("OldNumber"=w559) -> ("NewNumber"=w558:dbl)  [unwired: 1 in]
            n384 = property class="DigNum (严格)"(reference=w560, "Val(Sgnl)"=w558) -> ()  [unwired: 1 in, 2 out]
          }
          frame "Disabled and Grayed Out" {
            n385 = One Button Dialog(message="关闭连接后才可设置!" ("消息")) -> ()  [unwired: 1 in, 1 out]
          }
          frame "Disabled", Default {
            n386 = One Button Dialog(message="当前操作权限不足,请提升权限!!!" ("消息")) -> ()  [unwired: 1 in, 1 out]
          }
        }
      }
      event "密码锁": Value Change {
        n387 = event-data() -> ("NewVal"=w564:bool)  [unwired: 1 in, 5 out]
        n388 = case shown="假" w564 {
          frame False {
            n389 = global write "多参数全局变量.vi" "权限"(enum16{"一级权限", "二级权限", "三级权限"}."一级权限" ("权限")) -> ()
          }
          frame True {
            n390 = call "数字键盘.vi"("显示样式"=u32 2) -> ("NewNumber"=w569:dbl)  [unwired: 1 in]
            n391 = case shown="23506" w569 {
              tunnel: ["密码错误,即将切换为一级权限!" ("Infoin") "密码正确,即将切换为二级权限!" ("Infoin") "密码正确,即将切换为三级权限!" ("Infoin")] -> w568
              tunnel: [u32 16711680 ("颜色盒") _ _] -> w567
              tunnel: [enum16{"一级权限", "二级权限", "三级权限"}."一级权限" ("权限") enum16{"一级权限", "二级权限", "三级权限"}."二级权限" ("权限") enum16{"一级权限", "二级权限", "三级权限"}."三级权限" ("权限")] -> w566
              frame 0, Default {
              }
              frame 666 {
              }
              frame 23506 {
              }
            }
            n392 = global write "多参数全局变量.vi" "权限"(w566) -> ()
            n393 = call "TimeLmtDialog.vi"("颜色盒"=w567, "Infoin"=w568) -> ()  [unwired: 10 in]
          }
        }
      }
      event "周期设置": Mouse Down {
        n394 = event-data() -> ()  [unwired: 1 in, 6 out]
        n395 = flat-sequence {
          frame #0 {
            n396 = global read "断电保存变量.vi" "定时控制输入"() -> (w579:T15)
            n397 = call "周期设置.vi"("定时控制输入"=w579) -> ("定时控制输出"=w578:T15)  [unwired: 10 in]
            n398 = global write "断电保存变量.vi" "定时控制输入"(w578) -> ()
          }
          frame #1 {
            n399 = call "配置文件保存.vi"() -> ()  [unwired: 12 in]
          }
        }
      }
      event "水样测试": Value Change {
        n400 = event-data() -> ()  [unwired: 1 in, 6 out]
        n401 = vi-ref "水样测试.vi"() -> (w583:refnum<vi>)
        n402 = property class="VI"(reference=w583) -> ("Name"=w587:string, "Exec.State"=w585:T16)  [unwired: 1 in, 2 out]
        n403 = Open VI Reference(type specifier VI Refnum (for type only)=refnum<vi> refnum, vi path=w587, options=128 ("选项")) -> (vi reference=w588:refnum<vi>)  [unwired: 3 in, 1 out]
        n404 = global read "多参数全局变量.vi" "运行模式"() -> (w581:enum16{"维护模式", "常规模式", "应急模式", "质控模式"})
        n405 = case shown="\"常规模式\", 默认" w581 {
          tunnel: ["M" ("数据标记表") "hd" ("数据标记表")] -> w580
          frame "维护模式" {
          }
          frame "常规模式", Default {
          }
        }
        n406 = case shown="\"Idle\"" w585 {
          tunnel: [w591 w594] -> w584
          tunnel: w588 -> [w591 w593]
          tunnel: w580 -> [_ w592]
          frame "Bad", Default {
          }
          frame "Idle" {
            n407 = call-by-ref "开始异步调用"(reference=w593, "数据标记表"=w592) -> (reference out=w594:refnum<vi>)  [unwired: 12 in, 1 out]
          }
        }
        n408 = Close Reference(reference=w584) -> ()  [unwired: 1 in, 1 out]
      }
      event "标样核查": Value Change {
        n409 = event-data() -> ()  [unwired: 1 in, 6 out]
        n410 = call "标样核查配置.vi"() -> ("确认输出"=w595:bool)  [unwired: 11 in]
        n411 = case shown="真" w595 {
          frame False {
          }
          frame True {
            n412 = vi-ref "标样核查.vi"() -> (w597:refnum<vi>)
            n413 = property class="VI"(reference=w597) -> ("Name"=w601:string, "Exec.State"=w599:T16)  [unwired: 1 in, 2 out]
            n414 = Open VI Reference(type specifier VI Refnum (for type only)=refnum<vi> refnum, vi path=w601, options=128 ("选项")) -> (vi reference=w602:refnum<vi>)  [unwired: 3 in, 1 out]
            n415 = case shown="\"Idle\"" w599 {
              tunnel: [w603 w605] -> w598
              tunnel: w602 -> [w603 w604]
              frame "Bad", Default {
              }
              frame "Idle" {
                n416 = call-by-ref "开始异步调用"(reference=w604) -> (reference out=w605:refnum<vi>)  [unwired: 13 in, 1 out]
              }
            }
            n417 = Close Reference(reference=w598) -> ()  [unwired: 1 in, 1 out]
          }
        }
      }
      event "停止": Value Change {
        w606 = u16 3 items=["空闲", "水样测试", "标样核查", "停止"] ("主副屏同步启动")
        n418 = event-data() -> ()  [unwired: 1 in, 6 out]
        n419 = Send Notification(notification=TRUE ("通知"), notifier=w608) -> ()  [unwired: 1 in, 2 out]
        n420 = global write "多参数全局变量.vi" "主副屏同步启动"(w606) -> ()
      }
      event "设置": Value Change {
        n421 = event-data() -> ()  [unwired: 1 in, 6 out]
        n422 = property on="窗格" class="Pane"("Origin"=T3 {"Horizontal"=0, "Vertical"=628} ("原点")) -> ()  [unwired: 2 in, 2 out]
      }
      event "仪器参数": Value Change {
        n423 = event-data() -> ()  [unwired: 1 in, 6 out]
        n424 = global read "断电保存变量.vi" "叶绿素参数"() -> (w610:T10)
        n425 = global read "断电保存变量.vi" "藻密度参数"() -> (w611:T10)
        n426 = global read "断电保存变量.vi" "电导率参数"() -> (w618:T10)
        n427 = global read "断电保存变量.vi" "溶解氧参数"() -> (w616:T10)
        n428 = global read "断电保存变量.vi" "ORP参数"() -> (w612:T10)
        n429 = global read "断电保存变量.vi" "水温参数"() -> (w619:T10)
        n430 = global read "断电保存变量.vi" "浊度参数"() -> (w617:T10)
        n431 = global read "断电保存变量.vi" "PH参数"() -> (w620:T10)
        n432 = Build Array(w620, w619, w618, w616, w617, w610, w611, w612) -> (w615:T22)
        n433 = call "仪器参数设置.vi"("仪器参数设置输入"=w615) -> ("确定"=w614:bool, "仪器参数设置输出"=w613:T22)  [unwired: 9 in]
        n434 = case shown="真" w614 {
          tunnel: w613 -> [_ w621]
          frame False {
          }
          frame True {
            n435 = flat-sequence {
              tunnel: w621 -> [w630]
              frame #0 {
                n436 = Index Array(array=w630) -> (element #1=w628:T10, element #2=w627:T10, element #3=w625:T10, element #4=w626:T10, element #5=w629:T10, element #6=w624:T10, element #7=w622:T10, element #8=w623:T10)  [unwired: 8 in]
                n437 = global write "断电保存变量.vi" "叶绿素参数"(w624) -> ()
                n438 = global write "断电保存变量.vi" "藻密度参数"(w622) -> ()
                n439 = global write "断电保存变量.vi" "PH参数"(w628) -> ()
                n440 = global write "断电保存变量.vi" "水温参数"(w627) -> ()
                n441 = global write "断电保存变量.vi" "电导率参数"(w625) -> ()
                n442 = global write "断电保存变量.vi" "溶解氧参数"(w626) -> ()
                n443 = global write "断电保存变量.vi" "浊度参数"(w629) -> ()
                n444 = global write "断电保存变量.vi" "ORP参数"(w623) -> ()
              }
              frame #1 {
                n445 = call "配置文件保存.vi"() -> ()  [unwired: 12 in]
              }
            }
          }
        }
      }
      event "pH", "DO", "Turb", "Cond", "Temp", "叶绿素a启用", "藻密度", "VISA资源名称", "连接方式", "IP", "Port", "自动断线重连", "ORP启用", "水样稳定时间", "水样保存组数", "COD启用": Value Change {
        n446 = event-data() -> ()  [unwired: 1 in, 6 out]
        n447 = flat-sequence {
          frame #0 {
            n448 = global write "断电保存变量.vi" "IP"("IP") -> ()
            n449 = global write "断电保存变量.vi" "藻密度"("藻密度") -> ()
            n450 = global write "断电保存变量.vi" "连接方式"("连接方式") -> ()
            n451 = global write "断电保存变量.vi" "Temp"("Temp") -> ()
            n452 = global write "断电保存变量.vi" "DO"("DO") -> ()
            n453 = global write "断电保存变量.vi" "Turb"("Turb") -> ()
            n454 = global write "断电保存变量.vi" "Port"("Port") -> ()
            n455 = global write "断电保存变量.vi" "pH"("pH") -> ()
            n456 = global write "断电保存变量.vi" "orp"("ORP启用") -> ()
            n457 = global write "断电保存变量.vi" "Cond"("Cond") -> ()
            n458 = global write "断电保存变量.vi" "水样测试组数"("水样保存组数") -> ()
            n459 = global write "断电保存变量.vi" "叶绿素a启用"("叶绿素a启用") -> ()
            n460 = global write "断电保存变量.vi" "VISA资源名称"("VISA资源名称") -> ()
            n461 = global write "断电保存变量.vi" "水样稳定时间"("水样稳定时间") -> ()
            n462 = local read "自动断线重连"() -> (w635:bool)
            n463 = global write "断电保存变量.vi" "COD"("COD启用") -> ()
            n464 = global write "断电保存变量.vi" "自动断线重连"(w635) -> ()
          }
          frame #1 {
            n465 = call "配置文件保存.vi"() -> ()  [unwired: 12 in]
          }
          frame #2 {
          }
        }
      }
      event "打开modbus": Value Change {
        n466 = event-data() -> ()  [unwired: 1 in, 6 out]
        n467 = global read "多参数全局变量.vi" "MB session in"() -> (w653:refnum<class "MB_Master.lvclass">)
        n468 = Flush Queue(queue=w648) -> (queue out=w647:refnum<queue>)  [unwired: 1 in, 2 out]
        n469 = property class="MB_Master"(reference=w653) -> ("Properties:Session Valid"=w652:bool)  [unwired: 1 in, 2 out]
        n470 = Select(t="close" ("元素"), s=w652, f="open" ("元素")) -> (s? t:f=w649:string)
        n471 = Enqueue Element(queue=w647, element=w649) -> ()  [unwired: 2 in, 3 out]
      }
      event "探头校正返回", "设置页返回": Value Change {
        n472 = event-data() -> ()  [unwired: 1 in, 6 out]
        n473 = property on="窗格" class="Pane"("Origin"=T3 {"Horizontal"=0, "Vertical"=0} ("原点")) -> ()  [unwired: 2 in, 2 out]
      }
      event "探头校正", "校准选择.水温校准": Value Change {
        n474 = event-data() -> ()  [unwired: 1 in, 6 out]
        n475 = property on="窗格" class="Pane"("Origin"=T3 {"Horizontal"=1656, "Vertical"=0} ("原点")) -> ()  [unwired: 2 in, 2 out]
        n476 = vi-ref "水温校准.vi"() -> (w655:refnum<vi>)
        n477 = property class="VI"(reference=w655) -> (reference out=w657:refnum<vi>, "Exec.State"=w656:T16)  [unwired: 1 in, 1 out]
        n478 = case shown="\"Bad\", 默认" w656 {
          tunnel: [w661 w663] -> w659
          tunnel: w657 -> [w661 w662]
          frame "Bad", Default {
          }
          frame "Idle" {
            n479 = invoke class="VI" method="Run VI"(reference=w662, "Wait until done"=FALSE ("结束前等待"), "Auto Dispose Ref"=FALSE ("自动销毁引用")) -> (reference out=w663:refnum<vi>)  [unwired: 2 in, 4 out]
          }
        }
        n480 = invoke on="探头校准子面板" class="SubPnl" method="Remove VI"() -> (error out=w658:errorcluster)  [unwired: 3 in, 2 out]
        n481 = invoke on="探头校准子面板" class="SubPnl" method="Insert VI"(error in=w658, "VI Ref"=w659) -> ()  [unwired: 2 in, 4 out]
      }
      event "校准选择.pH校准": Value Change {
        n482 = event-data() -> ()  [unwired: 1 in, 6 out]
        n483 = global read "断电保存变量.vi" "探头选择"() -> (w671:T13)
        n484 = Unbundle By Name(w671) -> ("pH探头选择"=w670:u16)
        n485 = case shown="2" w670 {
          tunnel: [w675 w676 w677] -> w669
          frame 0, Default {
            n486 = vi-ref "斯坦道多参数.lvlib:禹山pH校准.vi"() -> (w675:refnum<vi>)
          }
          frame 1 {
            n487 = vi-ref "斯坦道多参数.lvlib:pH电极校准.vi"() -> (w676:refnum<vi>)
          }
          frame 2 {
            n488 = vi-ref "斯坦道多参数.lvlib:纳清pH电极校准.vi"() -> (w677:refnum<vi>)
          }
        }
        n489 = property class="VI"(reference=w669) -> (reference out=w673:refnum<vi>, "Exec.State"=w672:T16)  [unwired: 1 in, 1 out]
        n490 = case shown="\"Bad\", 默认" w672 {
          tunnel: w673 -> [w678 w682]
          tunnel: [w678 w679] -> w667
          frame "Bad", Default {
          }
          frame "Idle" {
            n491 = invoke class="VI" method="Run VI"(reference=w682, "Wait until done"=FALSE ("结束前等待"), "Auto Dispose Ref"=FALSE ("自动销毁引用")) -> (reference out=w679:refnum<vi>)  [unwired: 2 in, 4 out]
          }
        }
        n492 = global read "多参数全局变量.vi" "校准VI引用句柄"() -> (w668:T21)
        n493 = invoke on="探头校准子面板" class="SubPnl" method="Remove VI"() -> (error out=w674:errorcluster)  [unwired: 3 in, 2 out]
        n494 = invoke on="探头校准子面板" class="SubPnl" method="Insert VI"(error in=w674, "VI Ref"=w667) -> ()  [unwired: 2 in, 4 out]
        n495 = Bundle By Name(cluster=w668, "pH校准VI引用句柄"=w667) -> (w666:T21)
        n496 = global write "多参数全局变量.vi" "校准VI引用句柄"(w666) -> ()
      }
      event "校准选择.电导率校准": Value Change {
        n497 = event-data() -> ()  [unwired: 1 in, 6 out]
        n498 = global read "断电保存变量.vi" "探头选择"() -> (w688:T13)
        n499 = Unbundle By Name(w688) -> ("电导率探头选择"=w687:u16)
        n500 = case shown="2" w687 {
          tunnel: [w692 w693 w694] -> w686
          frame 0, Default {
            n501 = vi-ref "斯坦道多参数.lvlib:禹山电导率校准.vi"() -> (w692:refnum<vi>)
          }
          frame 1 {
            n502 = vi-ref "斯坦道多参数.lvlib:电导率电极校准.vi"() -> (w693:refnum<vi>)
          }
          frame 2 {
            n503 = vi-ref "斯坦道多参数.lvlib:纳清电导率电极校准.vi"() -> (w694:refnum<vi>)
          }
        }
        n504 = property class="VI"(reference=w686) -> (reference out=w690:refnum<vi>, "Exec.State"=w689:T16)  [unwired: 1 in, 1 out]
        n505 = case shown="\"Bad\", 默认" w689 {
          tunnel: [w695 w697] -> w683
          tunnel: w690 -> [w695 w696]
          frame "Bad", Default {
          }
          frame "Idle" {
            n506 = invoke class="VI" method="Run VI"(reference=w696, "Wait until done"=FALSE ("结束前等待"), "Auto Dispose Ref"=FALSE ("自动销毁引用")) -> (reference out=w697:refnum<vi>)  [unwired: 2 in, 4 out]
          }
        }
        n507 = global read "多参数全局变量.vi" "校准VI引用句柄"() -> (w685:T21)
        n508 = invoke on="探头校准子面板" class="SubPnl" method="Remove VI"() -> (error out=w691:errorcluster)  [unwired: 3 in, 2 out]
        n509 = Bundle By Name(cluster=w685, "COND校准VI引用句柄"=w683) -> (w684:T21)
        n510 = invoke on="探头校准子面板" class="SubPnl" method="Insert VI"(error in=w691, "VI Ref"=w683) -> ()  [unwired: 2 in, 4 out]
        n511 = global write "多参数全局变量.vi" "校准VI引用句柄"(w684) -> ()
      }
      event "校准选择.溶解氧校准": Value Change {
        n512 = event-data() -> ()  [unwired: 1 in, 6 out]
        n513 = global read "断电保存变量.vi" "探头选择"() -> (w705:T13)
        n514 = Unbundle By Name(w705) -> ("DO探头选择"=w704:u16)
        n515 = case shown="2" w704 {
          tunnel: [w709 w710 w711] -> w703
          frame 0, Default {
            n516 = vi-ref "斯坦道多参数.lvlib:禹山溶解氧校准.vi"() -> (w709:refnum<vi>)
          }
          frame 1 {
            n517 = vi-ref "斯坦道多参数.lvlib:溶解氧电极校准.vi"() -> (w710:refnum<vi>)
          }
          frame 2 {
            n518 = vi-ref "斯坦道多参数.lvlib:纳清DO电极校准.vi"() -> (w711:refnum<vi>)
          }
        }
        n519 = property class="VI"(reference=w703) -> (reference out=w707:refnum<vi>, "Exec.State"=w706:T16)  [unwired: 1 in, 1 out]
        n520 = case shown="\"Bad\", 默认" w706 {
          tunnel: [w712 w714] -> w700
          tunnel: w707 -> [w712 w713]
          frame "Bad", Default {
          }
          frame "Idle" {
            n521 = invoke class="VI" method="Run VI"(reference=w713, "Wait until done"=FALSE ("结束前等待"), "Auto Dispose Ref"=FALSE ("自动销毁引用")) -> (reference out=w714:refnum<vi>)  [unwired: 2 in, 4 out]
          }
        }
        n522 = global read "多参数全局变量.vi" "校准VI引用句柄"() -> (w702:T21)
        n523 = invoke on="探头校准子面板" class="SubPnl" method="Remove VI"() -> (error out=w708:errorcluster)  [unwired: 3 in, 2 out]
        n524 = invoke on="探头校准子面板" class="SubPnl" method="Insert VI"(error in=w708, "VI Ref"=w700) -> ()  [unwired: 2 in, 4 out]
        n525 = Bundle By Name(cluster=w702, "DO校准VI引用句柄"=w700) -> (w701:T21)
        n526 = global write "多参数全局变量.vi" "校准VI引用句柄"(w701) -> ()
      }
      event "校准选择.浊度校准": Value Change {
        n527 = event-data() -> ()  [unwired: 1 in, 6 out]
        n528 = global read "断电保存变量.vi" "探头选择"() -> (w722:T13)
        n529 = Unbundle By Name(w722) -> ("浊度探头选择"=w721:u16)
        n530 = case shown="2" w721 {
          tunnel: [w726 w727 w728] -> w720
          frame 0, Default {
            n531 = vi-ref "斯坦道多参数.lvlib:禹山浊度校准.vi"() -> (w726:refnum<vi>)
          }
          frame 1 {
            n532 = vi-ref "斯坦道多参数.lvlib:浊度电极校准.vi"() -> (w727:refnum<vi>)
          }
          frame 2 {
            n533 = vi-ref "斯坦道多参数.lvlib:纳清浊度电极校准.vi"() -> (w728:refnum<vi>)
          }
        }
        n534 = property class="VI"(reference=w720) -> (reference out=w724:refnum<vi>, "Exec.State"=w723:T16)  [unwired: 1 in, 1 out]
        n535 = case shown="\"Bad\", 默认" w723 {
          tunnel: [w729 w731] -> w717
          tunnel: w724 -> [w729 w730]
          frame "Bad", Default {
          }
          frame "Idle" {
            n536 = invoke class="VI" method="Run VI"(reference=w730, "Wait until done"=FALSE ("结束前等待"), "Auto Dispose Ref"=FALSE ("自动销毁引用")) -> (reference out=w731:refnum<vi>)  [unwired: 2 in, 4 out]
          }
        }
        n537 = global read "多参数全局变量.vi" "校准VI引用句柄"() -> (w719:T21)
        n538 = invoke on="探头校准子面板" class="SubPnl" method="Remove VI"() -> (error out=w725:errorcluster)  [unwired: 3 in, 2 out]
        n539 = invoke on="探头校准子面板" class="SubPnl" method="Insert VI"(error in=w725, "VI Ref"=w717) -> ()  [unwired: 2 in, 4 out]
        n540 = Bundle By Name(cluster=w719, "TURB校准VI引用句柄"=w717) -> (w718:T21)
        n541 = global write "多参数全局变量.vi" "校准VI引用句柄"(w718) -> ()
      }
      event "校准选择.叶绿素a校准": Value Change {
        n542 = event-data() -> ()  [unwired: 1 in, 6 out]
        n543 = global read "断电保存变量.vi" "探头选择"() -> (w738:T13)
        n544 = Unbundle By Name(w738) -> ("叶绿素a探头选择"=w737:u16)
        n545 = case shown="2" w737 {
          tunnel: [w743 _ w744] -> w739
          frame 0, Default {
            n546 = vi-ref "禹山叶绿素a校准.vi"() -> (w743:refnum<vi>)
          }
          frame 1 {
          }
          frame 2 {
            n547 = vi-ref "斯坦道多参数.lvlib:纳清叶绿素a电极校准.vi"() -> (w744:refnum<vi>)
          }
        }
        n548 = property class="VI"(reference=w739) -> (reference out=w741:refnum<vi>, "Exec.State"=w740:T16)  [unwired: 1 in, 1 out]
        n549 = case shown="\"Bad\", 默认" w740 {
          tunnel: [w745 w747] -> w734
          tunnel: w741 -> [w745 w746]
          frame "Bad", Default {
          }
          frame "Idle" {
            n550 = invoke class="VI" method="Run VI"(reference=w746, "Wait until done"=FALSE ("结束前等待"), "Auto Dispose Ref"=FALSE ("自动销毁引用")) -> (reference out=w747:refnum<vi>)  [unwired: 2 in, 4 out]
          }
        }
        n551 = global read "多参数全局变量.vi" "校准VI引用句柄"() -> (w736:T21)
        n552 = invoke on="探头校准子面板" class="SubPnl" method="Remove VI"() -> (error out=w742:errorcluster)  [unwired: 3 in, 2 out]
        n553 = invoke on="探头校准子面板" class="SubPnl" method="Insert VI"(error in=w742, "VI Ref"=w734) -> ()  [unwired: 2 in, 4 out]
        n554 = Bundle By Name(cluster=w736, "CHLA校准VI引用句柄"=w734) -> (w735:T21)
        n555 = global write "多参数全局变量.vi" "校准VI引用句柄"(w735) -> ()
      }
      event "校准选择.藻密度校准": Value Change {
        n556 = event-data() -> ()  [unwired: 1 in, 6 out]
        n557 = global read "断电保存变量.vi" "探头选择"() -> (w754:T13)
        n558 = Unbundle By Name(w754) -> ("蓝绿藻探头选择"=w753:u16)
        n559 = case shown="2" w753 {
          tunnel: [_ w759] -> w755
          frame 0, Default {
          }
          frame 2 {
            n560 = vi-ref "斯坦道多参数.lvlib:纳清蓝绿藻电极校准.vi"() -> (w759:refnum<vi>)
          }
        }
        n561 = property class="VI"(reference=w755) -> (reference out=w757:refnum<vi>, "Exec.State"=w756:T16)  [unwired: 1 in, 1 out]
        n562 = case shown="\"Bad\", 默认" w756 {
          tunnel: [w760 w762] -> w750
          tunnel: w757 -> [w760 w761]
          frame "Bad", Default {
          }
          frame "Idle" {
            n563 = invoke class="VI" method="Run VI"(reference=w761, "Wait until done"=FALSE ("结束前等待"), "Auto Dispose Ref"=FALSE ("自动销毁引用")) -> (reference out=w762:refnum<vi>)  [unwired: 2 in, 4 out]
          }
        }
        n564 = global read "多参数全局变量.vi" "校准VI引用句柄"() -> (w752:T21)
        n565 = invoke on="探头校准子面板" class="SubPnl" method="Remove VI"() -> (error out=w758:errorcluster)  [unwired: 3 in, 2 out]
        n566 = invoke on="探头校准子面板" class="SubPnl" method="Insert VI"(error in=w758, "VI Ref"=w750) -> ()  [unwired: 2 in, 4 out]
        n567 = Bundle By Name(cluster=w752, "BGA校准VI引用句柄"=w750) -> (w751:T21)
        n568 = global write "多参数全局变量.vi" "校准VI引用句柄"(w751) -> ()
      }
      event "校准选择.ORP校准": Value Change {
        n569 = event-data() -> ()  [unwired: 1 in, 6 out]
        n570 = global read "断电保存变量.vi" "探头选择"() -> (w769:T13)
        n571 = Unbundle By Name(w769) -> ("orp探头选择"=w768:u16)
        n572 = case shown="1" w768 {
          tunnel: [_ w774] -> w770
          frame 0, Default {
          }
          frame 1 {
            n573 = vi-ref "斯坦道多参数.lvlib:ORP电极校准.vi"() -> (w774:refnum<vi>)
          }
        }
        n574 = property class="VI"(reference=w770) -> (reference out=w772:refnum<vi>, "Exec.State"=w771:T16)  [unwired: 1 in, 1 out]
        n575 = case shown="\"Bad\", 默认" w771 {
          tunnel: [w775 w777] -> w765
          tunnel: w772 -> [w775 w776]
          frame "Bad", Default {
          }
          frame "Idle" {
            n576 = invoke class="VI" method="Run VI"(reference=w776, "Wait until done"=FALSE ("结束前等待"), "Auto Dispose Ref"=FALSE ("自动销毁引用")) -> (reference out=w777:refnum<vi>)  [unwired: 2 in, 4 out]
          }
        }
        n577 = global read "多参数全局变量.vi" "校准VI引用句柄"() -> (w767:T21)
        n578 = invoke on="探头校准子面板" class="SubPnl" method="Remove VI"() -> (error out=w773:errorcluster)  [unwired: 3 in, 2 out]
        n579 = Bundle By Name(cluster=w767, "ORP校准VI引用句柄"=w765) -> (w766:T21)
        n580 = invoke on="探头校准子面板" class="SubPnl" method="Insert VI"(error in=w773, "VI Ref"=w765) -> ()  [unwired: 2 in, 4 out]
        n581 = global write "多参数全局变量.vi" "校准VI引用句柄"(w766) -> ()
      }
      event "校准选择.COD校准": Value Change {
        n582 = event-data() -> ()  [unwired: 1 in, 6 out]
        n583 = global read "断电保存变量.vi" "探头选择"() -> (w784:T13)
        n584 = Unbundle By Name(w784) -> ("COD探头选择"=w783:u16)
        n585 = case shown="1" w783 {
          tunnel: [_ w789] -> w785
          frame 0, Default {
          }
          frame 1 {
            n586 = vi-ref "斯坦道多参数.lvlib:COD电极校准.vi"() -> (w789:refnum<vi>)
          }
        }
        n587 = property class="VI"(reference=w785) -> (reference out=w787:refnum<vi>, "Exec.State"=w786:T16)  [unwired: 1 in, 1 out]
        n588 = case shown="\"Bad\", 默认" w786 {
          tunnel: [w790 w792] -> w780
          tunnel: w787 -> [w790 w791]
          frame "Bad", Default {
          }
          frame "Idle" {
            n589 = invoke class="VI" method="Run VI"(reference=w791, "Wait until done"=FALSE ("结束前等待"), "Auto Dispose Ref"=FALSE ("自动销毁引用")) -> (reference out=w792:refnum<vi>)  [unwired: 2 in, 4 out]
          }
        }
        n590 = global read "多参数全局变量.vi" "校准VI引用句柄"() -> (w782:T21)
        n591 = invoke on="探头校准子面板" class="SubPnl" method="Remove VI"() -> (error out=w788:errorcluster)  [unwired: 3 in, 2 out]
        n592 = Bundle By Name(cluster=w782, "COD校准VI引用句柄"=w780) -> (w781:T21)
        n593 = invoke on="探头校准子面板" class="SubPnl" method="Insert VI"(error in=w788, "VI Ref"=w780) -> ()  [unwired: 2 in, 4 out]
        n594 = global write "多参数全局变量.vi" "校准VI引用句柄"(w781) -> ()
      }
    }
  }
  n595 = property on="编号" class="Str"("Visible"=w27) -> ()  [unwired: 2 in, 2 out]
